vi "test_hashlib_sha256_hmac.vi"() -> (3 "all_passed":bool)   [LabVIEW 2019]
uses:
  hashlib/hashlib/hashlib.lvlib
panel:
  out "sha256":string[](array[string])
  out "passed":bool[](array[boolean])
  in  "test_cases":T1(array[cluster])
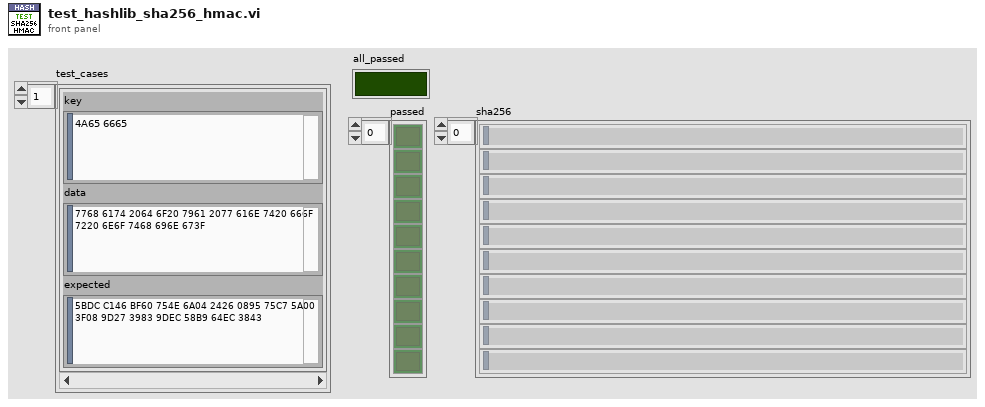
[diagram p1: front panel]
types:
  T1 = cluster{"key":string, "data":string, "expected":string}[]
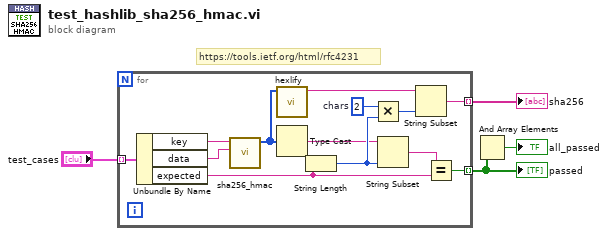
[diagram p0: block diagram]
diagram:
  # "https://tools.ietf.org/html/rfc4231"
  n1 = for {
    tunnel: "test_cases" -> [w17] mode=indexing
    tunnel: [w14] -> w3 mode=indexing
    tunnel: [w10] -> w1 mode=indexing
    w7 = 2  # chars
    n2 = Unbundle By Name(w17) -> ("key"=w16:string, "data"=w15:string, "expected"=w12:string)
    n3 = call "sha256_hmac.vi"("data"=w15, "key"=w16) -> ("sha256"=w13:u32[])  [unwired: 9 in]
    n4 = call "hexlify.vi"("sha256"=w13) -> ("hex (0-9a-f)"=w11:string)  [unwired: 10 in]
    n5 = Type Cast(x=w13) -> (*(type *) &x=w6:string)  [unwired: 1 in]
    n6 = String Length(string=w12) -> (length=w9:i32)
    n7 = Multiply(x=w7, y=w9) -> (x*y=w8:i32)
    n8 = String Subset(string=w6, length (rest)=w9) -> (substring=w5:string)  [unwired: 1 in]
    n9 = String Subset(string=w11, length (rest)=w8) -> (substring=w10:string)  [unwired: 1 in]
    n10 = Equal?(x=w5, y=w12) -> (x = y?=w14:bool)
  }
  "passed" <- w3
  "sha256" <- w1
  n11 = And Array Elements(Boolean array=w3) -> (logical AND=→"all_passed":bool)
